vi "Periodic Tasks.vi"   [LabVIEW 2014]
doc: "This VI runs in parallel to other tasks. It can contain as many user-defined periodic loops as you need. These can carry out PID or other sorts of timed response."
uses:
  <vilib>/Rock Robotics/SystemInterfaces/Utilities/FPGA_UtilitiesLED Source.ctl
  <vilib>/Rock Robotics/SystemInterfaces/Utilities/FPGA_UtilitiesLED State.ctl
  Robot Global Data.vi
  <vilib>/Rock Robotics/WPI/Solenoid/WPI_SolenoidValue.ctl
  <vilib>/Rock Robotics/WPI/Solenoid/WPI_SolenoidSetEnum.vi
  <vilib>/Rock Robotics/Network Tables/SD Read Boolean.vi
types:
  T1 = typedef "WPI_SolenoidValue.ctl" = enum16{"Off", "On", "Forward", "Reverse"}
  T2 = typedef "WPI_SolenoidDevRef.ctl" = cluster{"DevStatus":errorcluster, "Solenoid Module":T3, "Forward Solenoid Channel":T4, "Reverse Solenoid Channel":T4}
  T3 = typedef "FPGA_TypedefSolenoidModule.ctl" = enum16{"Solenoid Module 1", "Solenoid Module 2"}
  T4 = typedef "WPI_SolenoidChannel.ctl" = enum8{"Solenoid 1", "Solenoid 2", "Solenoid 3", "Solenoid 4", "Solenoid 5", "Solenoid 6", "Solenoid 7", "Solenoid 8", "Invalid"}
  T5 = typedef "WPI_MotorControlDeviceRef.ctl" = cluster{"DeviceStatus":errorcluster, "Type":enum16{"PWM", "CAN"}, "PWM":cluster{"Digital Module":T6, "PWM Channel":T7, "DeadBand":T8}, "CAN":cluster{"Device Number":u8, "Control Mode":T9, "Semaphore":T10, "Max Vout":dbl}, "Invert":bool, "TransformRef":T11, "InvTransformRef":T11}
  T6 = typedef "FPGA_TypedefDigitalModule.ctl" = enum16{"Digital Module 1", "Digital Module 2"}
  T7 = typedef "FPGA_DIOPWMChannel.ctl" = enum8{"PWM 1", "PWM 2", "PWM 3", "PWM 4", "PWM 5", "PWM 6", "PWM 7", "PWM 8", "PWM 9", "PWM 10", "Invalid"}
  T8 = typedef "WPI_PWMDeadband.ctl" = cluster{"Name":string, "maxPositivePwm":i32, "minPositivePwm":i32, "centerPwm":i32, "maxNegativePwm":i32, "minNegativePwm":i32, "angularRange":u16}
  T9 = typedef "WPI_CANJaguar_ControlMode.ctl" = enum8{"Percent VBus", "Current", "Speed", "Position", "Voltage"}
  T10 = typedef "Semaphore RefNum" = refnum<k1>
  T11 = typedef "WPI_PWMTransform_ConPane.ctl" = refnum<vi>
  T12 = typedef "FPGA_UtilitiesLED State.ctl" = enum16{"Off", "On", "Toggle"}
  T13 = typedef "FPGA_UtilitiesLED Source.ctl" = enum16{"User LED", "FPGA LED"}
  T14 = typedef "WPI_CompressorDevRef.ctl" = cluster{"DevStatus":errorcluster, "DigitalInputDevRef":T15, "RelayDevRef":T17}
  T15 = typedef "WPI_DigitalInputDevRef.ctl" = cluster{"DevStatus":errorcluster, "DIO Channel":T16, "Digital Module":T6}
  T16 = typedef "FPGA_DIOChannel.ctl" = enum8{"DIO 1", "DIO 2", "DIO 3", "DIO 4", "DIO 5", "DIO 6", "DIO 7", "DIO 8", "DIO 9", "DIO 10", "DIO 11", "DIO 12", "DIO 13", "DIO 14", "Invalid"}
  T17 = typedef "WPI_RelayDevRef.ctl" = cluster{"DevStatus":errorcluster, "Relay Channel":T18, "Digital Module":T6, "Relay Direction":T19}
  T18 = typedef "FPGA_DIORelayChannel.ctl" = enum8{"Relay 1", "Relay 2", "Relay 3", "Relay 4", "Relay 5", "Relay 6", "Relay 7", "Relay 8", "Invalid"}
  T19 = typedef "WPI_RelayDirection.ctl" = enum16{"Both directions", "Forward only", "Reverse only"}
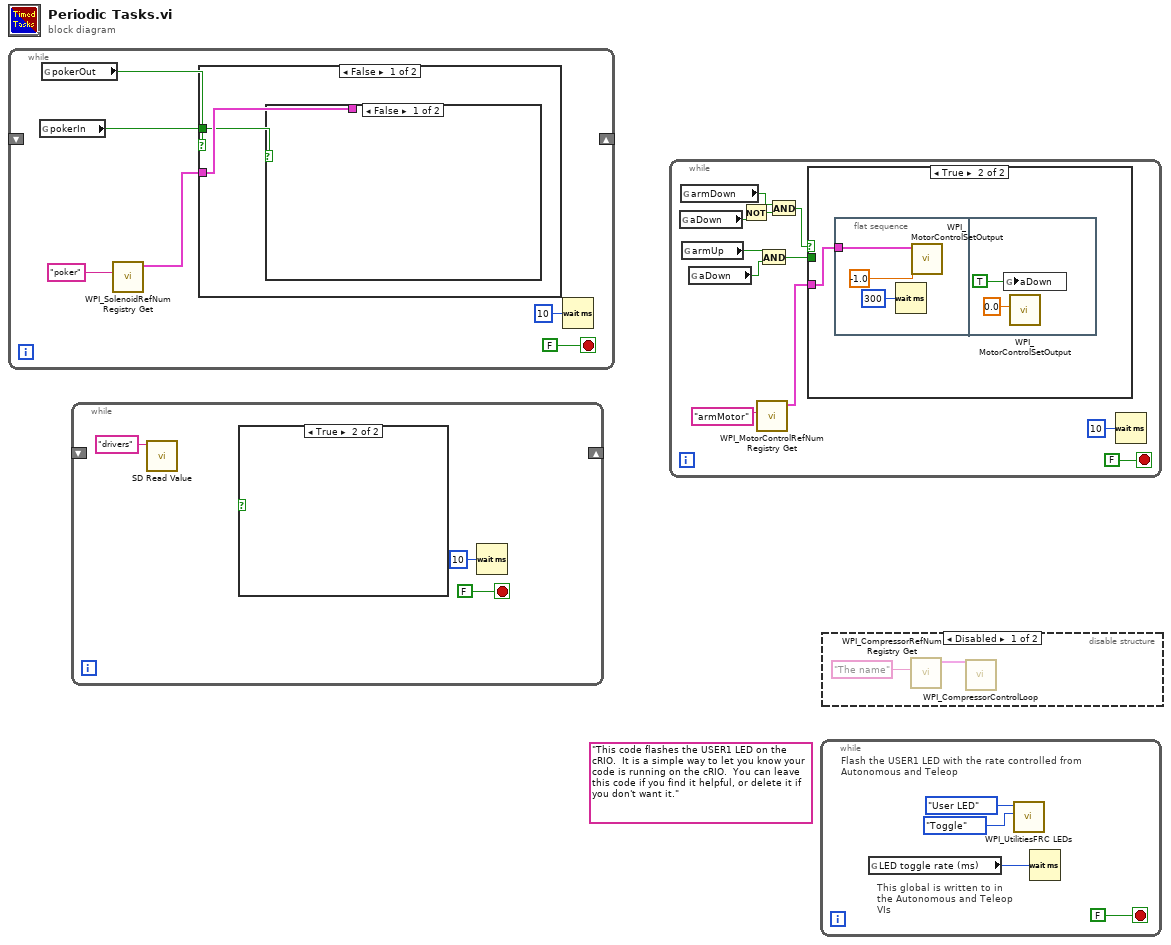
[diagram p0: block diagram]
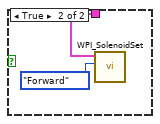
[diagram p3: hidden frame]
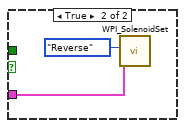
[diagram p4: hidden frame]
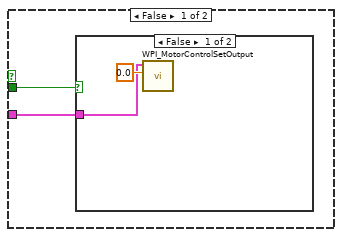
[diagram p5: hidden frame]
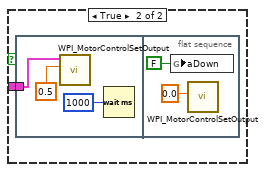
[diagram p6: hidden frame]
diagram:
  (unwired) "This code flashes the USER1 LED on the cRIO.  It is a simple way to let you know your code is running on the cRIO.  You can leave this code if you find it helpful, or delete it if you don't want it."
  n1 = while {
    shift-right: _ -> [_]
    shift-left: _ -> [_]
    stop <- FALSE stop-if-true
    n2 = global read "Robot Global Data.vi" "pokerIn"() -> (w3:bool)
    n3 = global read "Robot Global Data.vi" "pokerOut"() -> (w4:bool)
    n4 = call <vilib>:"WPI_SolenoidRefNum Registry Get.vi"("refnum name"="poker") -> ("SolenoidDevRef"=w1:T2)  [unwired: 9 in, 1 out]
    n5 = case shown="False" w4 {
      tunnel: w1 -> [w8 w11]
      tunnel: w3 -> [w7 _]
      frame False {
        n6 = case shown="False" w7 {
          tunnel: w8 -> [_ w10]
          frame False {
          }
          frame True {
            n7 = call-poly <vilib>:"WPI_SolenoidSet.vi"("Value"=WPI_SolenoidValue."Forward", "SolenoidDevRef"=w10) -> ()  [unwired: 8 in, 2 out]
          }
        }
      }
      frame True {
        n8 = call-poly <vilib>:"WPI_SolenoidSet.vi"("Value"=WPI_SolenoidValue."Reverse", "SolenoidDevRef"=w11) -> ()  [unwired: 8 in, 2 out]
      }
    }
    n9 = Wait (ms)(milliseconds to wait=u32 10) -> ()  [unwired: 1 out]
  }
  n10 = while {
    shift-right: _ -> [_]
    shift-left: _ -> [_]
    stop <- FALSE stop-if-true
    n11 = call-poly <vilib>:"SD Read Value.vi"("Name"="drivers") -> ()  [unwired: 8 in, 3 out]
    n12 = case shown="True" {
      selector: _ -> [_ _]
      frame False {
      }
      frame True {
      }
    }
    n13 = Wait (ms)(milliseconds to wait=u32 10) -> ()  [unwired: 1 out]
  }
  n14 = while {
    stop <- FALSE stop-if-true
    n15 = global read "Robot Global Data.vi" "aDown"() -> (w21:bool)
    n16 = global read "Robot Global Data.vi" "armDown"() -> (w20:bool)
    n17 = global read "Robot Global Data.vi" "armUp"() -> (w23:bool)
    n18 = global read "Robot Global Data.vi" "aDown"() -> (w24:bool)
    n19 = Not(x=w21) -> (.not. x?=w22:bool)
    n20 = call <vilib>:"WPI_MotorControlRefNum Registry Get.vi"("refnum name"="armMotor") -> ("MotorControlDevRef"=w16:T5)  [unwired: 9 in, 1 out]
    n21 = And(x=w23, y=w24) -> (x .and. y?=w17:bool)
    n22 = And(x=w20, y=w22) -> (x .and. y?=w18:bool)
    n23 = case shown="True" w18 {
      tunnel: w17 -> [w28 _]
      tunnel: w16 -> [w27 w37]
      frame False {
        n24 = case shown="False" w28 {
          tunnel: w27 -> [w29 w31]
          frame False {
            n25 = call <vilib>:"WPI_MotorControlSetOutput.vi"("Output"=0.0, "MotorControlDevRef"=w29) -> ()  [unwired: 7 in, 3 out]
          }
          frame True {
            n26 = flat-sequence {
              tunnel: w31 -> [w32]
              frame #0 {
                n27 = call <vilib>:"WPI_MotorControlSetOutput.vi"("Output"=0.5, "MotorControlDevRef"=w32) -> ()  [unwired: 7 in, 3 out]
                n28 = Wait (ms)(milliseconds to wait=u32 1000) -> ()  [unwired: 1 out]
              }
              frame #1 {
                n29 = global write "Robot Global Data.vi" "aDown"(FALSE ("aDown")) -> ()
                n30 = call <vilib>:"WPI_MotorControlSetOutput.vi"("Output"=0.0) -> ()  [unwired: 8 in, 3 out]
              }
            }
          }
        }
      }
      frame True {
        n31 = flat-sequence {
          tunnel: w37 -> [w38]
          frame #0 {
            n32 = Wait (ms)(milliseconds to wait=u32 300) -> ()  [unwired: 1 out]
            n33 = call <vilib>:"WPI_MotorControlSetOutput.vi"("Output"=-1.0, "MotorControlDevRef"=w38) -> ()  [unwired: 7 in, 3 out]
          }
          frame #1 {
            n34 = global write "Robot Global Data.vi" "aDown"(TRUE ("aDown")) -> ()
            n35 = call <vilib>:"WPI_MotorControlSetOutput.vi"("Output"=0.0) -> ()  [unwired: 8 in, 3 out]
          }
        }
      }
    }
    n36 = Wait (ms)(milliseconds to wait=u32 10) -> ()  [unwired: 1 out]
  }
  n37 = while {
    stop <- FALSE stop-if-true
    # "This global is written to in the Autonomous and Teleop VIs"
    # "Flash the USER1 LED with the rate controlled from Autonomous and Teleop"
    n38 = global read "Robot Global Data.vi" "LED toggle rate (ms)"() -> (w43:u32)
    n39 = call <vilib>:"WPI_UtilitiesFRC LEDs.vi"("State"=FPGA_UtilitiesLED_State."Toggle", "LED Type"=FPGA_UtilitiesLED_Source."User LED") -> ()  [unwired: 1 in, 9 out]
    n40 = Wait (ms)(milliseconds to wait=w43) -> ()  [unwired: 1 out]
  }
  n41 = disable-structure shown="Disabled" {
    frame Disabled {
      n42 = call <vilib>:"WPI_CompressorRefNum Registry Get.vi"("refnum name"="The name") -> ("CompressorDevRef"=w48:T14)  [unwired: 9 in, 1 out]
      n43 = call <vilib>:"WPI_CompressorControlLoop.vi"("CompressorDevRef"=w48) -> ()  [unwired: 11 in]
    }
    frame Enabled {
    }
  }
